vi "subvi_4.vi"(6 "error in (no error)":errorcluster, 9 "Continue":bool, 10 "password in":string, 11 "login in":string) -> (2 "password out":string, 3 "login out":string, 4 "error out":errorcluster)   [LabVIEW 2020]
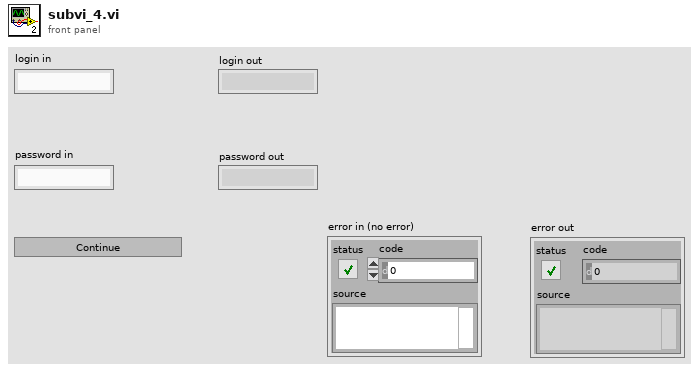
[diagram p1: front panel]
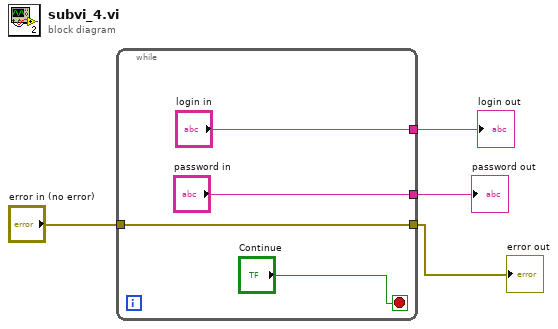
[diagram p0: block diagram]
diagram:
  n1 = while {
    tunnel: ["password in"] -> w3
    tunnel: ["login in"] -> w4
    tunnel: "error in (no error)" -> [w5]
    tunnel: [w5] -> w1
    stop <- "Continue" stop-if-true
  }
  "login out" <- w4
  "password out" <- w3
  "error out" <- w1
